vi "RPi_I2C_Read_Auto-Incrementing.vi"(0 "LINX Resource in":T1, 1 "I2C Channel (0)":u8, 2 "I2C Slave Address (0)":u8 format="%02x", 5 "Start Register Address":u8 format="%02x", 7 "Number of Bytes To Read":u8, 11 "error in (no error)":errorcluster) -> (4 "LINX Resource out":T1, 6 "Registers (Bytes)":u8[](array[numeric]), 15 "error out":errorcluster)   [LabVIEW 2020]
doc: "This procedure reads multiple registers from a I2C device that has the \"auto-incrementing\".\n\n<b>Start Register Address</b>\n the register address from which the reading begins\n<b>Number of Bytes To Read</b>\n the number of multiple consecutive register addresses to read.\n\nMIT License\nCopyright (c) 2021 Asper"
uses:
  <vilib>/MakerHub/LINX/Private/Type Defs/LINX Ref.ctl
  <vilib>/MakerHub/LINX/Private/Type Defs/Platform.ctl
  <vilib>/MakerHub/LINX/Private/Type Defs/Interface.ctl
  <vilib>/MakerHub/LINX/Private/Device/Type Defs/LINX Device Config.ctl
  <vilib>/MakerHub/LINX/Private/Device/Type Defs/TCP Config.ctl
  <vilib>/MakerHub/LINX/Private/Device/Type Defs/Channels.ctl
  <vilib>/MakerHub/LINX/Private/Local IO/LinxI2cWrite.vi
  <vilib>/MakerHub/LINX/Public/Utilities/Check Channel.vi
  <vilib>/MakerHub/LINX/Private/Local IO/Handle Errors.vi
  <vilib>/MakerHub/LINX/Private/Utilties/Generate Error.vi
  <vilib>/MakerHub/LINX/LMH-LINX.lvlib
  <vilib>/MakerHub/LINX/Private/Device/Device.lvlib
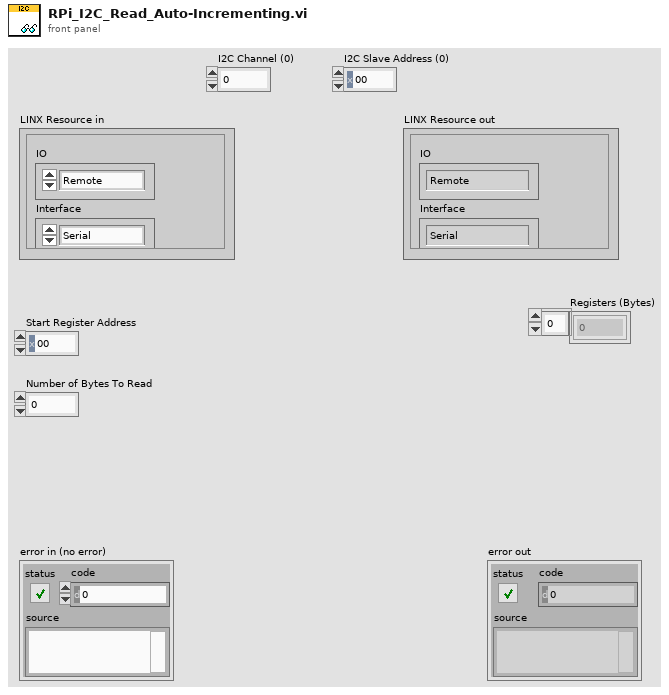
[diagram p1: front panel]
types:
  T1 = typedef "LMH-LINX.lvlib/LINX Ref.ctl" = cluster{"IO":T2, "Interface":T3, "LINX Device Config":T4}
  T2 = typedef "LMH-LINX.lvlib/Platform.ctl" = enum16{"Remote", "Local"}
  T3 = typedef "LMH-LINX.lvlib/Interface.ctl" = enum16{"Serial", "TCP"}
  T4 = typedef "LMH-LINX.lvlib/Device.lvlib/LINX Device Config.ctl" = cluster{"Interface":T3, "COM Port":refnum<visa-resource-name>, "TCP Configuration":T5, "Device Family":u8, "Device ID":u8, "Device Name":string, "TCP Ref":refnum<k5>, "Channels":T6}
  T5 = typedef "LMH-LINX.lvlib/Device.lvlib/TCP Config.ctl" = cluster{"IP Address":string, "Port":u16}
  T6 = typedef "LMH-LINX.lvlib/Channels.ctl" = cluster{"DI":u8[], "DO":u8[], "AI":u8[], "AO":u8[], "PWM":u8[], "QE":u8[], "UART":u8[], "I2C 2":u8[], "SPI":u8[], "CAN":u8[], "Servo":u8[], "AI Ref (V)":dbl, "AI Resolution (Bits)":u8, "AO Ref (V)":dbl, "AO Resolution (Bits)":u8}
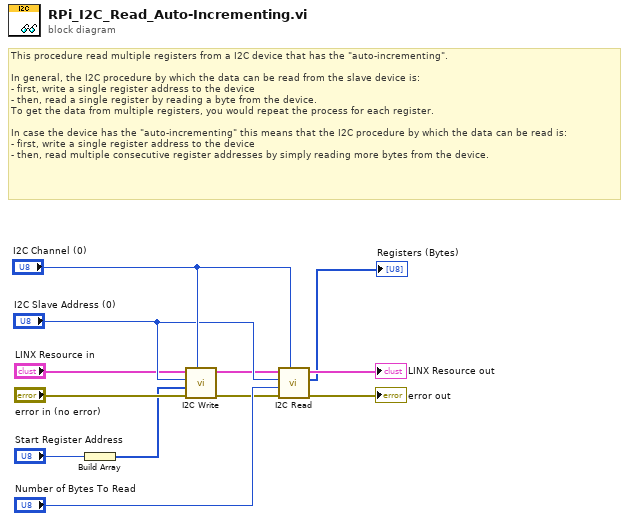
[diagram p0: block diagram]
diagram:
  # "This procedure read multiple registers from a I2C device that has the \"auto-incrementing\".\n\nIn general, the I2C procedure by which the data can be read from the slave device is:\n- first, write a single register address to the device\n- then, read a single register by reading a byte from the device.\nTo get the data from multiple registers, you would repeat the process for each register.\n\nIn case the device has the \"auto-incrementing\" this means that the I2C procedure by which the data can be read is:\n- first, write a single register address to the device\n- then, read multiple consecutive register addresses by simply reading more bytes from the device."
  n1 = Build Array("Start Register Address") -> (w2:u8[])
  n2 = call <vilib>:"I2C Write.vi"("I2C Channel"="I2C Channel (0)", "Error In"="error in (no error)", "Data"=w2, "I2C Slave Address (0)"="I2C Slave Address (0)", "LINX Resource"="LINX Resource in") -> ("Error Out"=w6:errorcluster, "LINX Resource"=w4:T1)  [unwired: 5 in]
  n3 = call <vilib>:"I2C Read.vi"("I2C Channel"="I2C Channel (0)", "Error In"=w6, "Bytes To Read"="Number of Bytes To Read", "I2C Slave Address (0)"="I2C Slave Address (0)", "LINX Resource"=w4) -> ("Error Out"=→"error out":errorcluster, "Data"=→"Registers (Bytes)":u8[], "LINX Resource"=→"LINX Resource out":T1)  [unwired: 4 in]
